vi "Execute Cmd.vi"() -> ()   [LabVIEW 2018]
uses:
  AltonTech MALT200817.lvlib
panel:
  out "Response":string
  in  "Request":string="SAY_HELLO_WOLRD"
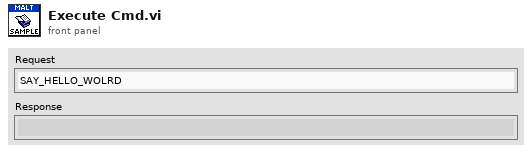
[diagram p1: front panel]
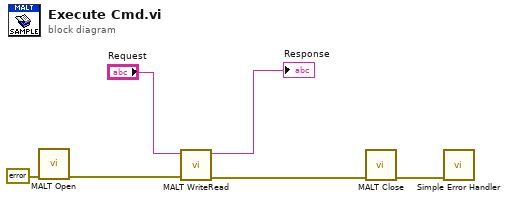
[diagram p0: block diagram]
diagram:
  n1 = call "MALT Open.vi"("error in"=errorcluster {"status"=FALSE, "code"=0, "source"=""}) -> ("error out"=w4:errorcluster)  [unwired: 10 in]
  n2 = call "MALT WriteRead.vi"("error in"=w4, "Request"="Request") -> ("error out"=w3:errorcluster, "Response"=→"Response":string)  [unwired: 8 in]
  n3 = call "MALT Close.vi"("error in"=w3) -> ("error out"=w2:errorcluster)  [unwired: 10 in]
  n4 = call <vilib>:"Simple Error Handler.vi"("error in (no error)"=w2) -> ()  [unwired: 4 in, 5 out]
